vi "Generate DAQ Link Message.vi"(2 "error in":errorcluster, 3 "All Data":dbl[](array[numeric])) -> (0 "error out":errorcluster, 1 "Message":string)   [LabVIEW 2009]
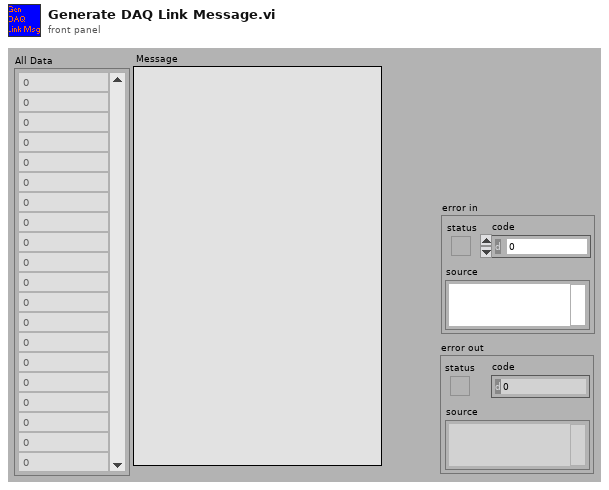
[diagram p1: front panel]
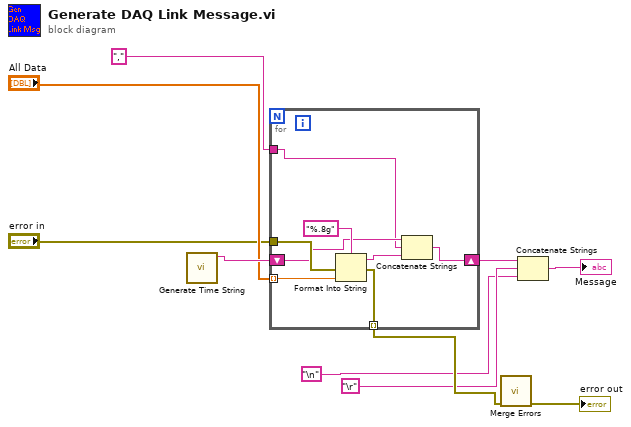
[diagram p0: block diagram]
diagram:
  n1 = call "Generate Time String.vi"() -> ("date/time string"=w10:string)  [unwired: 11 out]
  n2 = for {
    tunnel: "All Data" -> [w11] mode=indexing
    shift-right: [w16] -> w5
    shift-left: w10 -> [w13]
    tunnel: "error in" -> [w15]
    tunnel: [w14] -> w4 mode=indexing
    tunnel: "," -> [w12]
    n3 = Format Into String(format string="%.8g", error in=w15, w11) -> (resulting string=w17:string, error out=w14:errorcluster)  [unwired: 1 in]
    n4 = Concatenate Strings(w13, w12, w17) -> (w16:string)
  }
  n5 = call <vilib>:"Merge Errors.vi"("error array in"=w4) -> ("error out"=→"error out":errorcluster)  [unwired: 3 in, 3 out]
  n6 = Concatenate Strings(w5, "\r", "\n") -> (→"Message":string)
